vi "Network Send.vi"(8 "error in (no error)":errorcluster, 10 "Target IP Address":string="localhost", 11 "Electrophysiology in":refnum<class "Behavior.lvclass">) -> (0 "error out":errorcluster, 3 "Electrophysiology out":refnum<class "Behavior.lvclass">)   [LabVIEW 2010]
uses:
  Behavior.lvclass
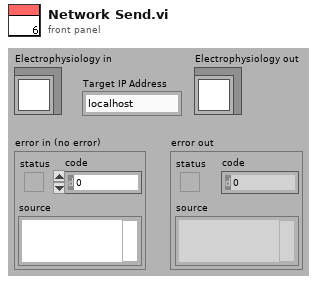
[diagram p1: front panel]
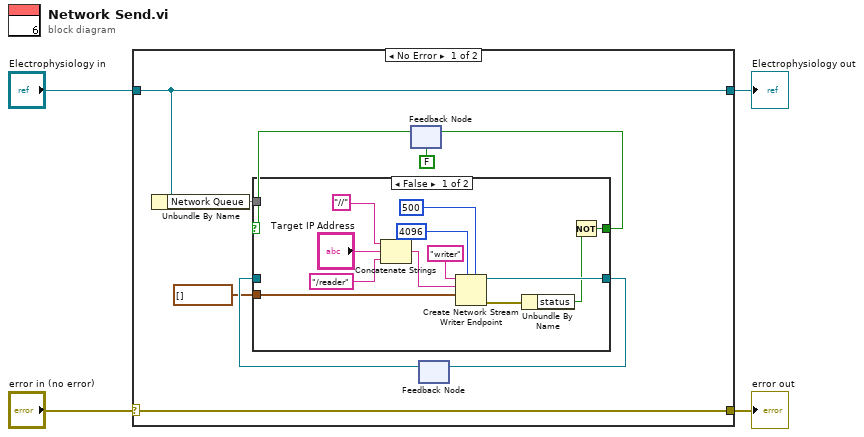
[diagram p0: block diagram]
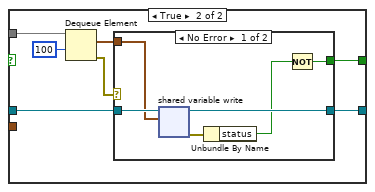
[diagram p2: hidden frame]
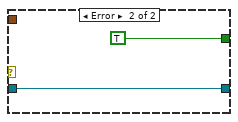
[diagram p3: hidden frame]
diagram:
  n1 = case shown="No Error" "error in (no error)" {
    selector: "error in (no error)" -> [w13 w42]
    tunnel: [w13 w42] -> w3
    tunnel: [w6 w41] -> w1
    tunnel: "Electrophysiology in" -> [w6 w41]
    frame No Error {
      n2 = Unbundle By Name(w6) -> ("Network Queue"=w5)
      n3 = feedback #1(FALSE) -> (w11:bool)
      n4 = feedback #2() -> (w9:refnum<k21>)  [unwired: 1 in]
      n5 = case shown="False" w11 {
        tunnel: waveform(dbl)[] [] -> [w22 _]
        tunnel: [w18 w26] -> w12
        tunnel: [w20 w29] -> w10
        tunnel: w9 -> [_ w31]
        tunnel: w5 -> [_ w32]
        frame False {
          n6 = Concatenate Strings("//" ("reader url"), "Target IP Address", "/reader" ("string")) -> (w14:string)
          n7 = Create Network Stream Writer Endpoint(5:500 ("timeout in ms (-1)"), 7:4096 ("writer buffer size"), 9:w22, 10:w14, 11:"writer" ("writer name")) -> (0:w21:errorcluster, 3:w20:refnum<k21>)  [unwired: 1 in]
          n8 = Unbundle By Name(w21) -> ("status"=w19:bool)
          n9 = Not(x=w19) -> (.not. x?=w18:bool)
        }
        frame True {
          n10 = Dequeue Element(queue=w32, timeout in ms (-1)=100) -> (element=w30:waveform(dbl)[], error out=w27:errorcluster)  [unwired: 1 in, 2 out]
          n11 = case shown="No Error" w27 {
            tunnel: w31 -> [w38 w40]
            tunnel: w30 -> [w37 _]
            tunnel: [w36 w40] -> w29
            tunnel: [w34 TRUE] -> w26
            frame No Error {
              n12 = shared-variable-write(w38, w37) -> (w36:refnum<k21>, w35:errorcluster)  [unwired: 2 in, 1 out]
              n13 = Unbundle By Name(w35) -> ("status"=w33:bool)
              n14 = Not(x=w33) -> (.not. x?=w34:bool)
            }
            frame Error {
            }
          }
        }
      }
      n15 = feedback-in #1(w12) -> ()
      n16 = feedback-in #2(w10) -> ()
    }
    frame Error {
    }
  }
  "error out" <- w3
  "Electrophysiology out" <- w1
